vi "Write Line to Std In .vi"(8 "error in":errorcluster, 10 "Input":string, 11 "ASE Handle":refnum<class "ase.lvclass">) -> (0 "error out":errorcluster, 1 "State":T1, 3 "ASE Handle Duplicate":refnum<class "ase.lvclass">)   [LabVIEW 2024, in "serenial.io-ase.lvlib" / "ase.lvclass"]
doc: "<B>Write a line to the standard input.</B>\n\nThis will append the newline \"\\n\" character to the end of any input\n\nThis VI generates the following errors:\n-5691000: Internal Library Error. Check Error Message for more details.\n1556: Invalid Handle Supplied"
uses:
  ase.lvclass
  Standard Input State.ctl
  ase.lvclass/ase.ctl
  Merge Call Library Errors.vi
  Error Invalid ASE Handle.vi
  Error Internal Library Implementation Error.vi
  <vilib>/Utility/error.llb/Error Cluster From Error Code.vi
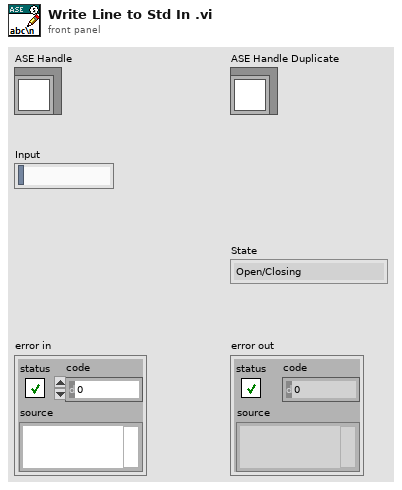
[diagram p1: front panel]
types:
  T1 = typedef "serenial.io-ase.lvlib/ase.lvclass/Standard Input State.ctl" = enum16{"Open/Closing", "Closed"}
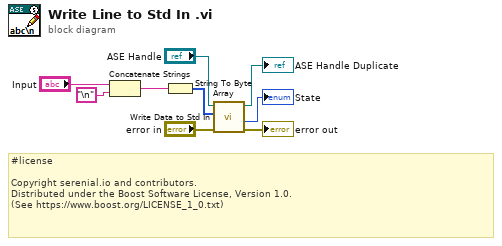
[diagram p0: block diagram]
diagram:
  # "#license\n\nCopyright serenial.io and contributors.\nDistributed under the Boost Software License, Version 1.0.\n(See https://www.boost.org/LICENSE_1_0.txt)"
  n1 = Concatenate Strings("Input", "\n") -> (w7:string)
  n2 = String To Byte Array(string=w7) -> (unsigned byte array=w6:u8[])
  n3 = call "Write Data to Std In.vi"("error in"="error in", "Data"=w6, "ASE Handle"="ASE Handle") -> ("error out"=→"error out":errorcluster, "State"=→"State":T1, "ASE Handle Duplicate"=→"ASE Handle Duplicate":refnum<class "ase.lvclass">)  [unwired: 6 in]
